vi "Draw.vi"(8 "error in (no error)":errorcluster, 9 "DrawPoint(Ingored If Not Wired)":T1={"X"=-1, "Y"=-1}, 10 "PictureIn":picture, 11 "reference in":refnum<class "Glyph.lvclass">) -> (0 "error out":errorcluster, 1 "Width":i32, 2 "PictureOut":picture, 3 "reference in":refnum<class "Glyph.lvclass">)   [LabVIEW 2012, in "Glyph.lvclass"]
uses:
  Glyph.lvclass
  Position.ctl
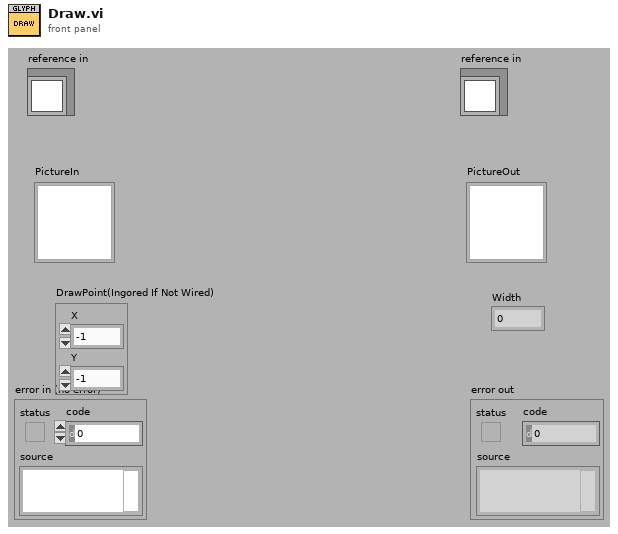
[diagram p1: front panel]
types:
  T1 = typedef "Glyph.lvclass/Position.ctl" = cluster{"X":i32, "Y":i32}
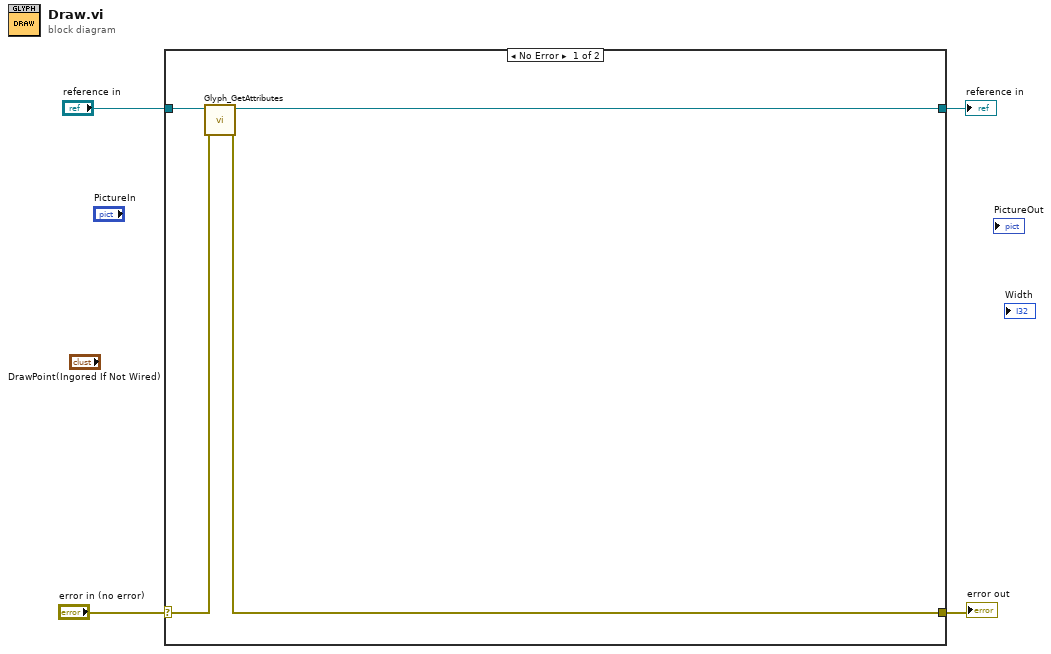
[diagram p0: block diagram]
diagram:
  n1 = case shown="No Error" "error in (no error)" {
    selector: "error in (no error)" -> [w8 w10]
    tunnel: [w7 w10] -> w3
    tunnel: [w5 w9] -> w1
    tunnel: "reference in" -> [w6 w9]
    frame No Error {
      n2 = call "Glyph_GetAttributes.vi"("error in (no error)"=w8, "reference in"=w6) -> ("error out"=w7:errorcluster, "reference out"=w5:refnum<class "Glyph.lvclass">)  [unwired: 6 in, 2 out]
    }
    frame Error {
    }
  }
  "error out" <- w3
  "reference in" <- w1
